vi "receive message.vi"(8 "error in (no error)":errorcluster, 11 "Socket in":refnum<class "Socket.lvclass">) -> (0 "error out":errorcluster, 3 "Socket out":refnum<class "Socket.lvclass">)   [LabVIEW 2018, in "Socket.lvclass"]
uses:
  Socket.lvclass
  Socket.lvclass/Socket.ctl
  <vilib>/addons/zeromq/zmq_socket.lvclass
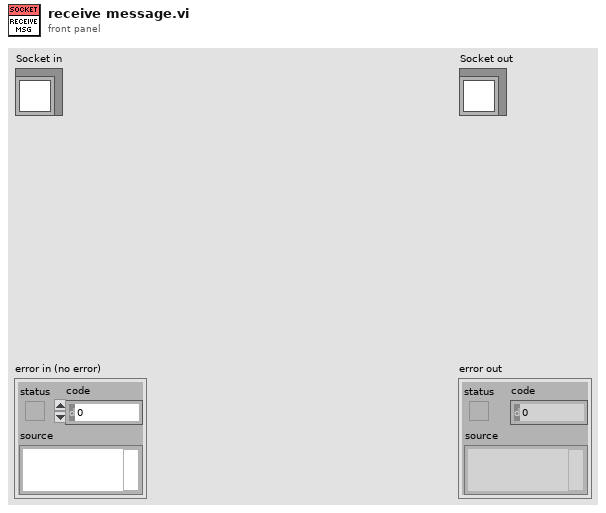
[diagram p1: front panel]
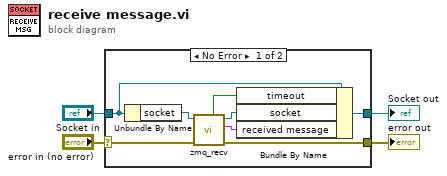
[diagram p0: block diagram]
diagram:
  n1 = case shown="No Error" "error in (no error)" {
    selector: "error in (no error)" -> [w12 w14]
    tunnel: [w11 w14] -> w3
    tunnel: [w8 w13] -> w1
    tunnel: "Socket in" -> [w9 w13]
    frame No Error {
      n2 = Unbundle By Name(w9) -> ("socket"=w10:refnum<class "zmq_socket.lvclass">)
      n3 = call <vilib>:"zmq_recv.vi"("error in"=w12, "socket in"=w10) -> ("error out"=w11:errorcluster, "data"=w6:string, "socket out"=w7:refnum<class "zmq_socket.lvclass">, "timeout?"=w5:bool)  [unwired: 3 in, 1 out]
      n4 = Bundle By Name(cluster=w9, "timeout"=w5, "socket"=w7, "received message"=w6) -> (w8:refnum<class "Socket.lvclass">)
    }
    frame Error {
    }
  }
  "error out" <- w3
  "Socket out" <- w1
